vi "Load Glyph.vi"(8 "error in (no error)":errorcluster, 10 "glyph_index":u32, 11 "face in":i64) -> (0 "error out":errorcluster, 3 "face out":i64)   [LabVIEW 2023, in "Freetype Drawer.lvlib"]
uses:
  Freetype Drawer.lvlib
  libfreetype.dll
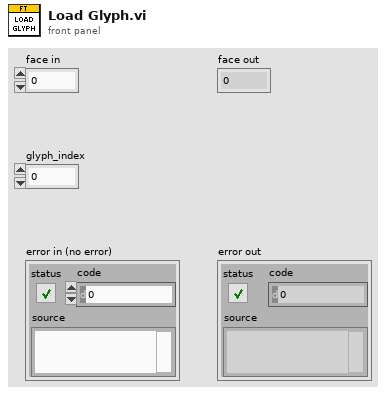
[diagram p1: front panel]
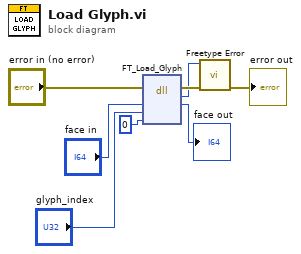
[diagram p0: block diagram]
diagram:
  n1 = dll-call lib="E:/Labview/LV 2023/Libs/LV Symbol/Freetype Drawer/libfreetype.dll" fn="FT_Load_Glyph"(error in="error in (no error)", "face"="face in", "glyph_index"="glyph_index", "load_flags"=0) -> (error out=w7:errorcluster, "error"=w6:i32, "face"=→"face out":i64)  [unwired: 4 in, 1 out]
  n2 = call "Freetype Error.vi"("error in (no error)"=w7, "Error"=w6) -> ("error out"=→"error out":errorcluster)  [unwired: 9 in]
